vi "Read Glyphs.vi"(8 "error in (no error)":errorcluster, 11 "LV Awesome in":refnum<class "LV Awesome.lvclass">) -> (0 "error out":errorcluster, 2 "Glyphs":map{string, u32}(c390), 3 "LV Awesome out":refnum<class "LV Awesome.lvclass">)   [LabVIEW 2023, in "LV-Awesome.lvlib" / "LV Awesome.lvclass"]
uses:
  LV Awesome.lvclass
  LV Awesome.lvclass/LV Awesome.ctl
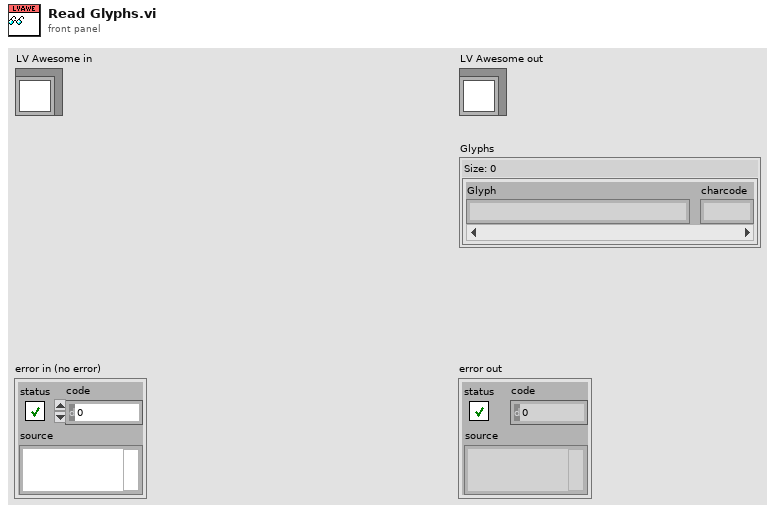
[diagram p1: front panel]
types:
  T1 = typedef "LV-Awesome.lvlib/LV Awesome.lvclass/Data.ctl" = cluster{"Glyphs":map{string, u32}, "Fonts":map{string, path}}
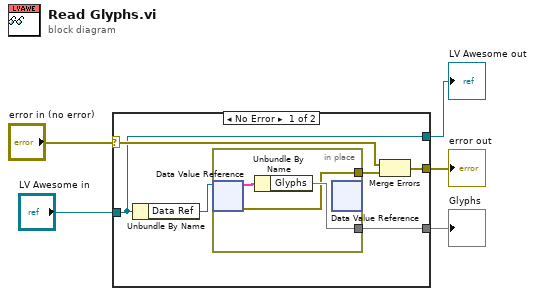
[diagram p0: block diagram]
diagram:
  n1 = case shown="No Error" "error in (no error)" {
    selector: "error in (no error)" -> [w11 w15]
    tunnel: [w7 w15] -> w3
    tunnel: [w10 w16] -> w2
    tunnel: "LV Awesome in" -> [w10 w16]
    tunnel: [w8 _] -> w1
    frame No Error {
      n2 = Unbundle By Name(w10) -> ("Data Ref"=w9:refnum<data-value>)
      n3 = in-place {
        in-place-border: [w13] -> w8
        in-place-border: [w12] -> w6
        n4 = in-place-dvr #1(w9) -> (w14:T1, w12:errorcluster)
        n5 = Unbundle By Name(w14) -> ("Glyphs"=w13:map{string, u32})
        n6 = in-place-dvr #1() -> ()  [unwired: 1 in, 2 out]
      }
      n7 = Merge Errors(w11, w6) -> (w7:errorcluster)
    }
    frame Error {
    }
  }
  "error out" <- w3
  "LV Awesome out" <- w2
  "Glyphs" <- w1
